vi "project vi.vi"() -> ()   [LabVIEW 2021]
panel:
  in  "a":dbl=1.0
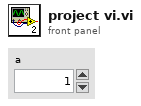
[diagram p1: front panel]
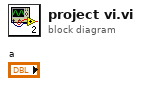
[diagram p0: block diagram]
diagram:
